vi "display_1s_stim_9s_ISI_CS1_CS2_no_trigger.vi"() -> ()   [LabVIEW 2019]
uses:
  <vilib>/Analysis/Matrix/Datatypes/RealMatrix.ctl
  <vilib>/Utility/file.llb/Write Delimited Spreadsheet (DBL).vi
  <vilib>/Analysis/Matrix/NI_Matrix.lvlib
panel:
  out "Num trials":u32=204
  out "ISI Time":dbl
  out "Stim TS":dbl
  out "Output":dbl[][](array[numeric])
  out "Output frame":T1
  out "Array temp1":T1
  out "Elapsed Time":dbl
  out "Display":bool=TRUE
  out "Trial":u32=1
  out "reward":dbl[](array[numeric])
  out "stim_id":dbl[](array[numeric])
  out "stim_loaded":dbl
  out "Timings":dbl[](array[numeric])
  out "Stimuli Loaded?":bool
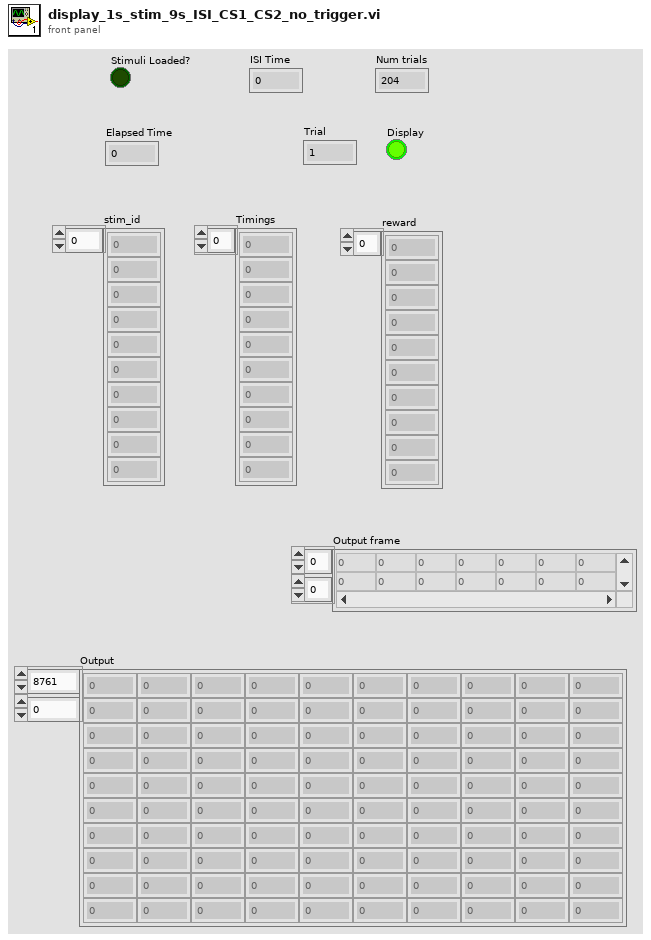
[diagram p1: front panel]
types:
  T1 = typedef "NI_Matrix.lvlib/RealMatrix.ctl" = dbl[][]
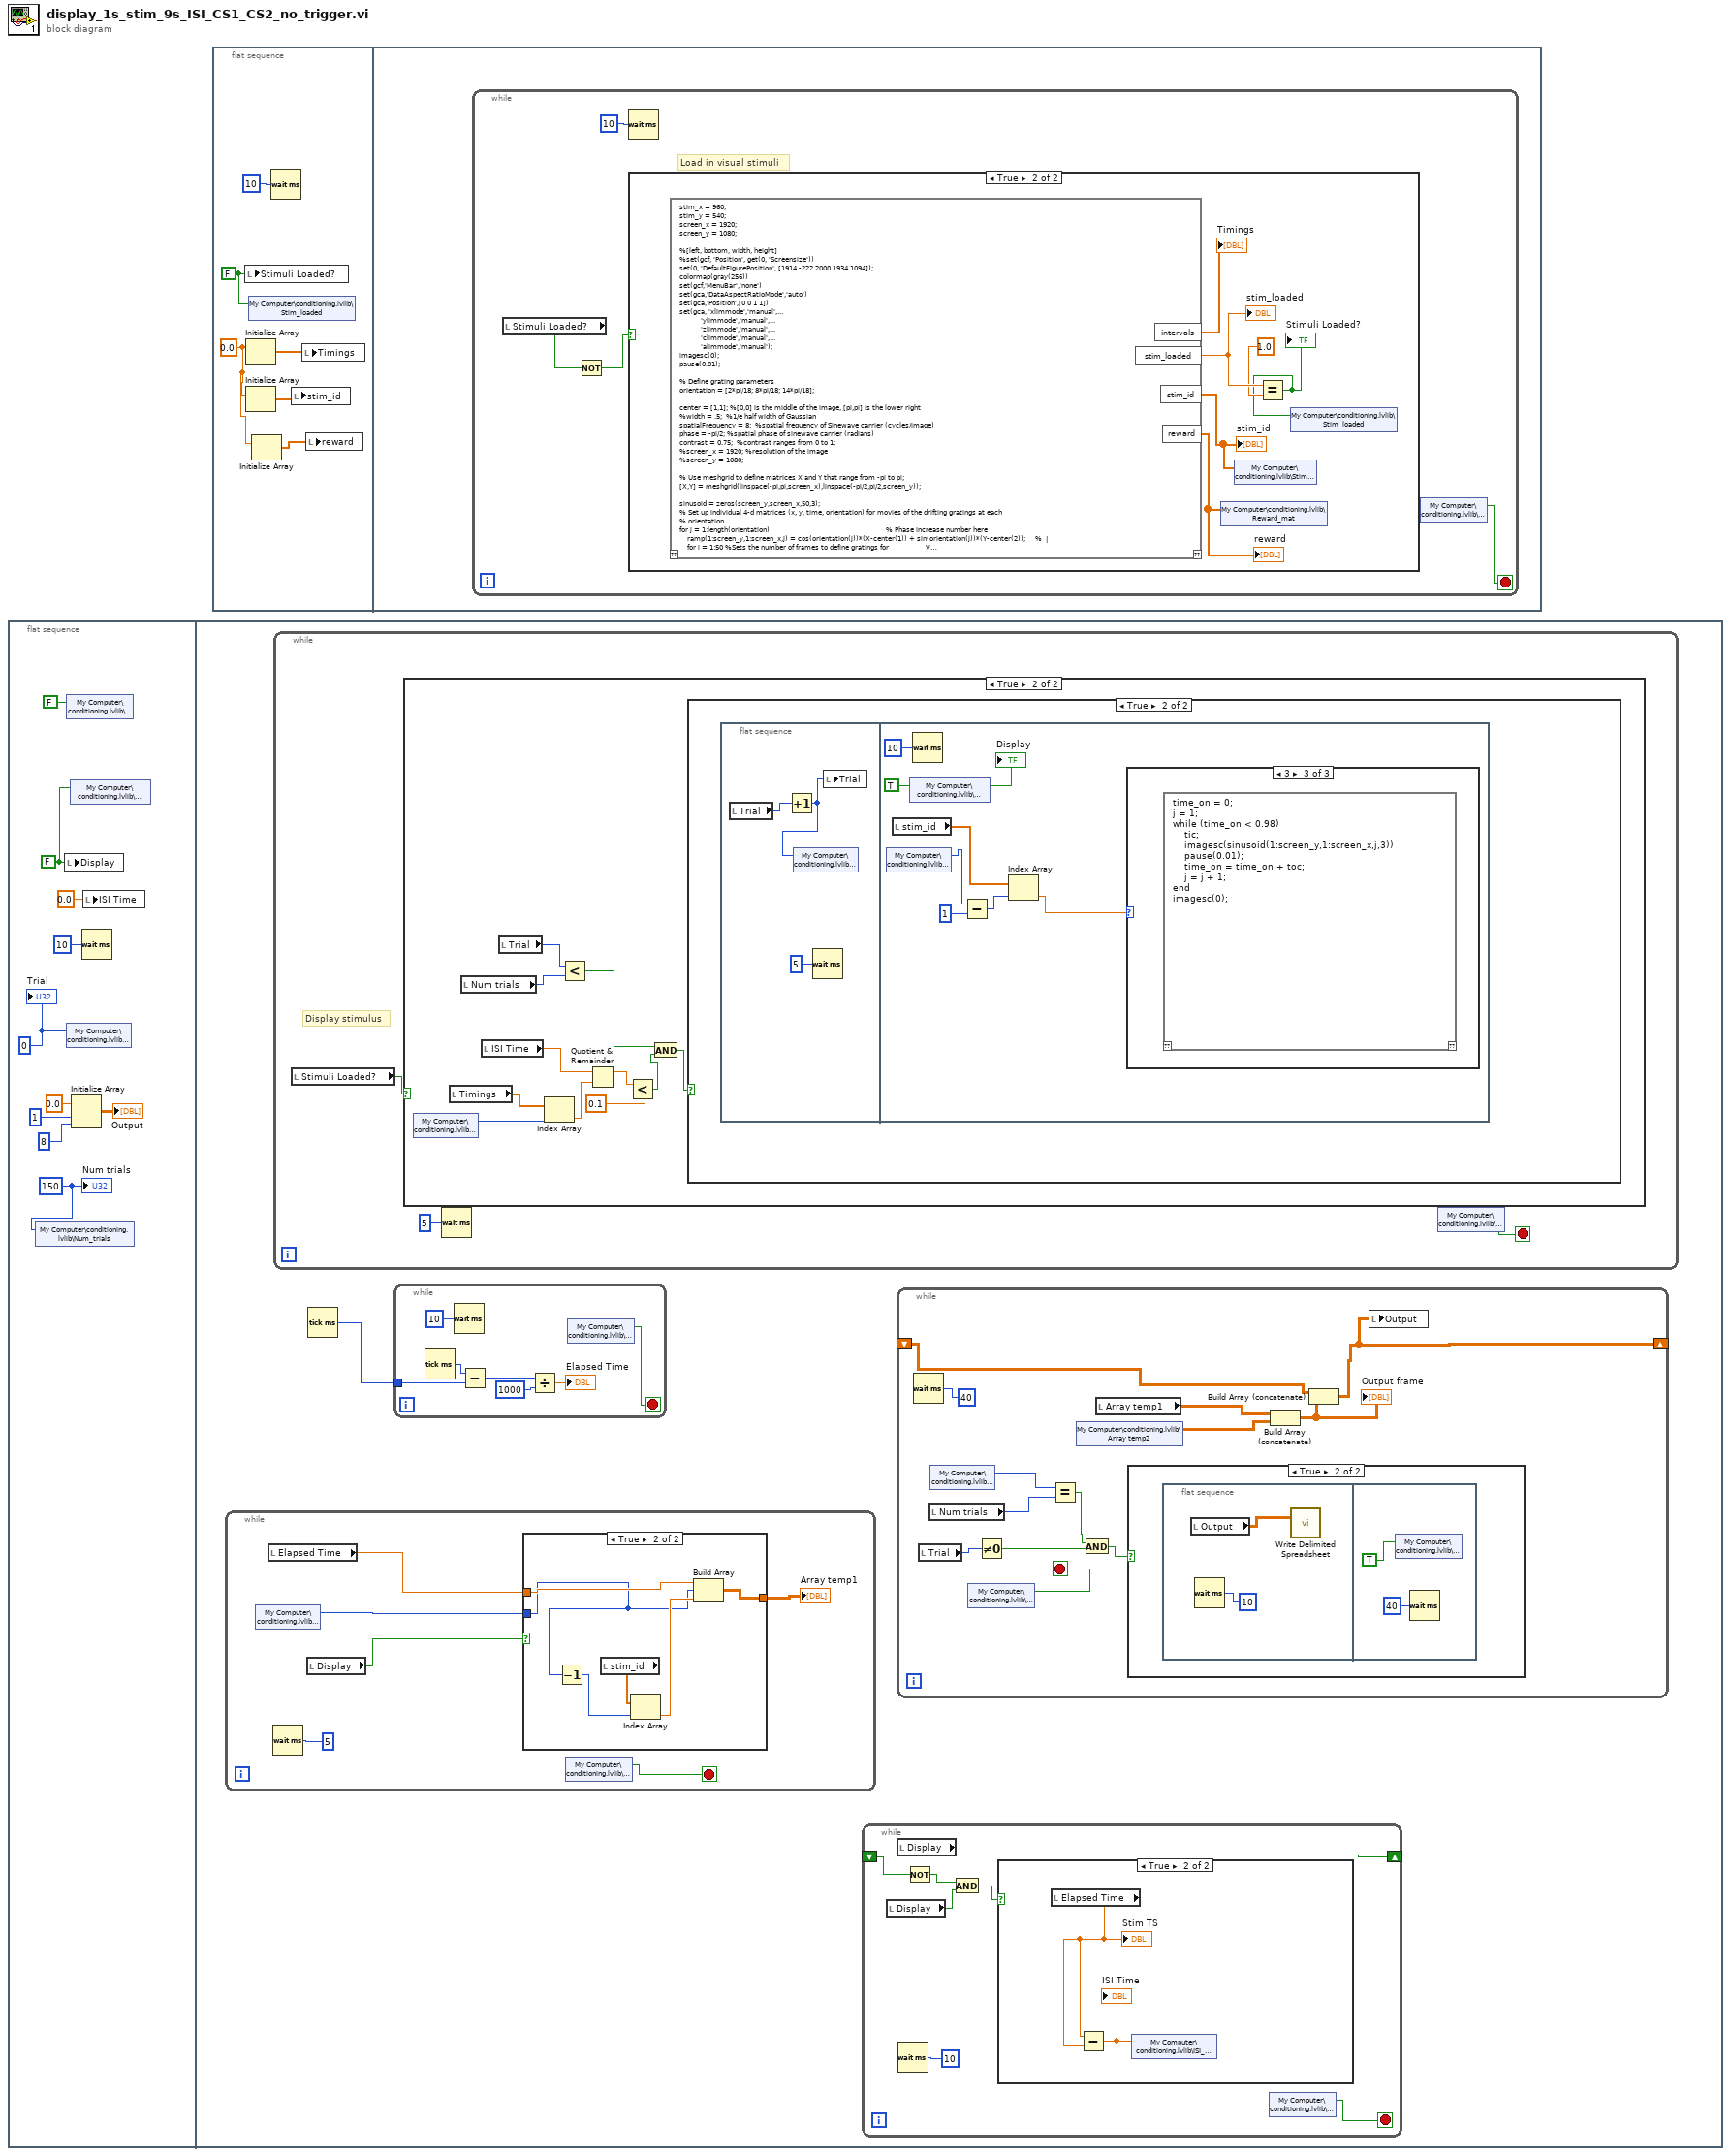
[diagram p0: block diagram]
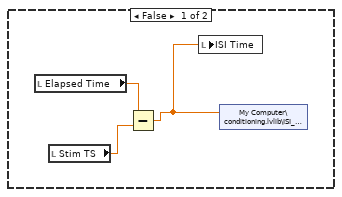
[diagram p3: hidden frame]
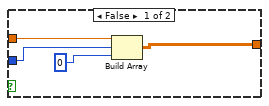
[diagram p4: hidden frame]
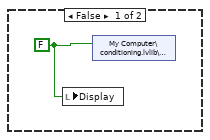
[diagram p7: hidden frame]
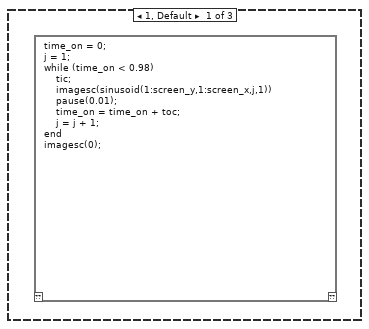
[diagram p8: hidden frame]
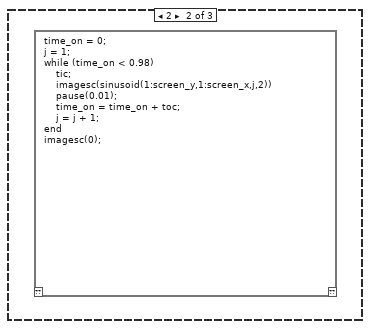
[diagram p9: hidden frame]
diagram:
  n1 = flat-sequence {
    frame #0 {
      w2 = u32 150
      w8 = FALSE ("Display")
      w10 = u32 0 ("Trial")
      n2 = shared-variable "My Computer\\conditioning.lvlib\\Num_trials"(w2) -> ()  [unwired: 1 in, 1 out]
      n3 = local write "Display"(w8) -> ()
      n4 = shared-variable "My Computer\\conditioning.lvlib\\Stop"(FALSE ("Stop")) -> ()  [unwired: 1 in, 1 out]
      n5 = shared-variable "My Computer\\conditioning.lvlib\\Trial"(w10) -> ()  [unwired: 1 in, 1 out]
      n6 = shared-variable "My Computer\\conditioning.lvlib\\Display"(w8) -> ()  [unwired: 1 in, 1 out]
      n7 = Initialize Array(0.0 ("element"), 1 ("dimension size"), 8 ("dimension size")) -> (→"Output":dbl[][])
      n8 = Wait (ms)(milliseconds to wait=u32 10) -> ()  [unwired: 1 out]
      n9 = local write "ISI Time"(0.0 ("ISI Time")) -> ()
      "Trial" <- w10
      "Num trials" <- w2
    }
    frame #1 {
      n10 = while {
        stop <- w24 stop-if-true
        n11 = shared-variable "My Computer\\conditioning.lvlib\\Trial"() -> (w26:u32)  [unwired: 1 in, 1 out]
        n12 = local read "Elapsed Time"() -> (w28:dbl)
        n13 = Wait (ms)(milliseconds to wait=u32 5) -> ()  [unwired: 1 out]
        n14 = local read "Display"() -> (w25:bool)
        n15 = case shown="True" w25 {
          tunnel: w26 -> [w32 w35]
          tunnel: w28 -> [w33 w37]
          tunnel: [w31 w38] -> w27
          frame False {
            n16 = Build Array(w33, w32, u32 0 ("milliseconds to wait")) -> (w31:T1)
          }
          frame True {
            n17 = Decrement(x=w35) -> (x-1=w34:u32)
            n18 = local read "stim_id"() -> (w39:dbl[])
            n19 = Index Array(array=w39, index=w34) -> (element=w36:dbl)
            n20 = Build Array(w37, w35, w36) -> (w38:T1)
          }
        }
        "Array temp1" <- w27
        n21 = shared-variable "My Computer\\conditioning.lvlib\\Stop"() -> (w24:bool)  [unwired: 1 in, 1 out]
      }
      n22 = while {
        stop <- w65 stop-if-true
        # "Display stimulus"
        n23 = local read "Stimuli Loaded?"() -> (w64:bool)
        n24 = case shown="True" w64 {
          frame False {
          }
          frame True {
            n25 = shared-variable "My Computer\\conditioning.lvlib\\Trial"() -> (w68:u32)  [unwired: 1 in, 1 out]
            n26 = local read "Timings"() -> (w75:dbl[])
            n27 = local read "Num trials"() -> (w67:u32)
            n28 = local read "ISI Time"() -> (w73:dbl)
            n29 = local read "Trial"() -> (w72:u32)
            n30 = Index Array(array=w75, index=w68) -> (element=w74:dbl)
            n31 = Less?(x=w72, y=w67) -> (x < y?=w71:bool)
            n32 = Quotient & Remainder(x=w73, y=w74) -> (x-y*floor(x/y)=w77:dbl)  [unwired: 1 out]
            n33 = Less?(x=w77, y=0.1) -> (x < y?=w70:bool)
            n34 = And(x=w71, y=w70) -> (x .and. y?=w69:bool)
            n35 = case shown="True" w69 {
              frame False {
                w78 = FALSE ("Display")
                n36 = local write "Display"(w78) -> ()
                n37 = shared-variable "My Computer\\conditioning.lvlib\\Display"(w78) -> ()  [unwired: 1 in, 1 out]
              }
              frame True {
                n38 = flat-sequence {
                  frame #0 {
                    n39 = local read "Trial"() -> (w80:u32)
                    n40 = Increment(x=w80) -> (x+1=w79:u32)
                    n41 = shared-variable "My Computer\\conditioning.lvlib\\Trial"(w79) -> ()  [unwired: 1 in, 1 out]
                    n42 = Wait (ms)(milliseconds to wait=u32 5) -> ()  [unwired: 1 out]
                    n43 = local write "Trial"(w79) -> ()
                  }
                  frame #1 {
                    w86 = TRUE ("Boolean")
                    n44 = shared-variable "My Computer\\conditioning.lvlib\\Trial"() -> (w84:u32)  [unwired: 1 in, 1 out]
                    n45 = local read "stim_id"() -> (w87:dbl[])
                    n46 = shared-variable "My Computer\\conditioning.lvlib\\Display"(w86) -> ()  [unwired: 1 in, 1 out]
                    n47 = Wait (ms)(milliseconds to wait=u32 10) -> ()  [unwired: 1 out]
                    n48 = Subtract(x=w84, y=u32 1) -> (x-y=w85:u32)
                    n49 = Index Array(array=w87, index=w85) -> (element=w82:dbl)
                    n50 = case shown="3" w82 {
                      frame 1, Default {
                        n51 = script code="time_on = 0;\nj = 1;\nwhile (time_on < 0.98)\n    tic;\n    imagesc(sinusoid(1:screen_y,1:screen_x,j,1))\n    pause(0.01);\n    time_on = time_on + toc;\n    j = j + 1;\nend\nimagesc(0);"() -> ()  [unwired: 1 in, 1 out]
                      }
                      frame 2 {
                        n52 = script code="time_on = 0;\nj = 1;\nwhile (time_on < 0.98)\n    tic;\n    imagesc(sinusoid(1:screen_y,1:screen_x,j,2))\n    pause(0.01);\n    time_on = time_on + toc;\n    j = j + 1;\nend\nimagesc(0);"() -> ()  [unwired: 1 in, 1 out]
                      }
                      frame 3 {
                        n53 = script code="time_on = 0;\nj = 1;\nwhile (time_on < 0.98)\n    tic;\n    imagesc(sinusoid(1:screen_y,1:screen_x,j,3))\n    pause(0.01);\n    time_on = time_on + toc;\n    j = j + 1;\nend\nimagesc(0);"() -> ()  [unwired: 1 in, 1 out]
                      }
                    }
                    "Display" <- w86
                  }
                }
              }
            }
          }
        }
        n54 = Wait (ms)(milliseconds to wait=u32 5) -> ()  [unwired: 1 out]
        n55 = shared-variable "My Computer\\conditioning.lvlib\\Stop"() -> (w65:bool)  [unwired: 1 in, 1 out]
      }
      n56 = Tick Count (ms)() -> (millisecond timer value=w11:u32)
      n57 = while {
        tunnel: w11 -> [w43]
        stop <- w40 stop-if-true
        n58 = Tick Count (ms)() -> (millisecond timer value=w44:u32)
        n59 = Wait (ms)(milliseconds to wait=u32 10) -> ()  [unwired: 1 out]
        n60 = Subtract(x=w44, y=w43) -> (x-y=w41:u32)
        n61 = Divide(x=w41, y=u32 1000) -> (x/y=→"Elapsed Time":dbl)
        n62 = shared-variable "My Computer\\conditioning.lvlib\\Stop"() -> (w40:bool)  [unwired: 1 in, 1 out]
      }
      n63 = while {
        shift-right: [w16] -> _
        shift-left: _ -> [w15]
        stop <- w18 stop-if-true
        n64 = local read "Display"() -> (w13:bool)
        n65 = local read "Display"() -> (w16:bool)
        n66 = Wait (ms)(milliseconds to wait=u32 10) -> ()  [unwired: 1 out]
        n67 = Not(x=w15) -> (.not. x?=w14:bool)
        n68 = And(x=w14, y=w13) -> (x .and. y?=w12:bool)
        n69 = case shown="True" w12 {
          frame False {
            n70 = local read "Elapsed Time"() -> (w19:dbl)
            n71 = local read "Stim TS"() -> (w21:dbl)
            n72 = Subtract(x=w19, y=w21) -> (x-y=w20:dbl)
            n73 = local write "ISI Time"(w20) -> ()
            n74 = shared-variable "My Computer\\conditioning.lvlib\\ISI_Time"(w20) -> ()  [unwired: 1 in, 1 out]
          }
          frame True {
            n75 = local read "Elapsed Time"() -> (w22:dbl)
            "Stim TS" <- w22
            n76 = Subtract(x=w22, y=w22) -> (x-y=w23:dbl)
            "ISI Time" <- w23
            n77 = shared-variable "My Computer\\conditioning.lvlib\\ISI_Time"(w23) -> ()  [unwired: 1 in, 1 out]
          }
        }
        n78 = shared-variable "My Computer\\conditioning.lvlib\\Stop"() -> (w18:bool)  [unwired: 1 in, 1 out]
      }
      n79 = while {
        shift-right: [w56] -> _
        shift-left: _ -> [w57]
        stop <- w59 stop-if-true
        n80 = Wait (ms)(milliseconds to wait=u32 40) -> ()  [unwired: 1 out]
        n81 = local read "Trial"() -> (w49:u32)
        n82 = local read "Num trials"() -> (w51:u32)
        n83 = shared-variable "My Computer\\conditioning.lvlib\\Trial"() -> (w52:u32)  [unwired: 1 in, 1 out]
        n84 = shared-variable "My Computer\\conditioning.lvlib\\Stop"() -> (w59:bool)  [unwired: 1 in, 1 out]
        n85 = Not Equal To 0?(x=w49) -> (x != 0?=w48:bool)
        n86 = Equal?(x=w52, y=w51) -> (x = y?=w50:bool)
        n87 = shared-variable "My Computer\\conditioning.lvlib\\Array temp2"() -> (w54:dbl[][])  [unwired: 1 in, 1 out]
        n88 = And(x=w50, y=w48) -> (x .and. y?=w47:bool)
        n89 = local read "Array temp1"() -> (w55:T1)
        n90 = case shown="True" w47 {
          frame False {
          }
          frame True {
            n91 = flat-sequence {
              frame #0 {
                n92 = local read "Output"() -> (w61:dbl[][])
                n93 = Wait (ms)(milliseconds to wait=u32 10) -> ()  [unwired: 1 out]
                n94 = call-poly <vilib>:"Write Delimited Spreadsheet.vi"("2D data"=w61) -> ()  [unwired: 13 in, 2 out]
              }
              frame #1 {
                n95 = shared-variable "My Computer\\conditioning.lvlib\\Stop"(TRUE) -> ()  [unwired: 1 in, 1 out]
                n96 = Wait (ms)(milliseconds to wait=u32 40) -> ()  [unwired: 1 out]
              }
            }
          }
        }
        n97 = Build Array (concatenate)(w55, w54) -> (w53:T1)
        "Output frame" <- w53
        n98 = Build Array (concatenate) ("Build Matrix")(w57, w53) -> (w56:T1)
        n99 = local write "Output"(w56) -> ()
      }
    }
  }
  n100 = flat-sequence {
    frame #0 {
      w91 = 0.0 ("element")
      w89 = FALSE ("Stimuli Loaded?")
      n101 = local write "Stimuli Loaded?"(w89) -> ()
      n102 = Initialize Array(w91) -> (w93:dbl[])  [unwired: 1 in]
      n103 = Initialize Array(w91) -> (w92:dbl[])  [unwired: 1 in]
      n104 = shared-variable "My Computer\\conditioning.lvlib\\Stim_loaded"(w89) -> ()  [unwired: 1 in, 1 out]
      n105 = Initialize Array(w91) -> (w90:dbl[])  [unwired: 1 in]
      n106 = Wait (ms)(milliseconds to wait=u32 10) -> ()  [unwired: 1 out]
      n107 = local write "stim_id"(w92) -> ()
      n108 = local write "Timings"(w93) -> ()
      n109 = local write "reward"(w90) -> ()
    }
    frame #1 {
      n110 = while {
        stop <- w97 stop-if-true
        # "Load in visual stimuli"
        n111 = local read "Stimuli Loaded?"() -> (w96:bool)
        n112 = Not(x=w96) -> (.not. x?=w95:bool)
        n113 = Wait (ms)(milliseconds to wait=u32 10) -> ()  [unwired: 1 out]
        n114 = case shown="True" w95 {
          frame False {
          }
          frame True {
            n115 = script code="stim_x = 960;\nstim_y = 540;\nscreen_x = 1920;\nscreen_y = 1080;\n\n%[left, bottom, width, height]\n%set(gcf, 'Position', get(0, 'Screensize'))\nset(0, 'DefaultFigurePosition', [1914 -222.2000 1934 1094]);\ncolormap(gray(256))\nset(gcf,'MenuBar','none')\nset(gca,'DataAspectRatioMode','auto')\nset(gca,'Position',[0 0 1 1])\nset(gca, 'xlimmode','manual',...\n           'ylimmode','manual',...\n           'zlimmode','manual',...\n           'climmode','manual',...\n           'alimmode','manual');\nimagesc(0);\npause(0.01);\n\n% Define grating parameters\norientation = [2*pi/18; 8*pi/18; 14*pi/18];\n\ncenter = [1,1]; %[0,0] is the middle of the image, [pi,pi] is the lower right\n%width = .5;  %1/e half width of Gaussian\nspatialFrequency = 8;  %spatial frequency of Sinewave carrier (cycles/image)\nphase = -pi/2; %spatial phase of sinewave carrier (radians)\ncontrast = 0.75;  %contrast ranges from 0 to 1;\n%screen_x = 1920; %resolution of the image  \n%screen_y = 1080;\n\n% Use meshgrid to define matrices X and Y that range from -pi to pi;\n[X,Y] = meshgrid(linspace(-pi,pi,screen_x),linspace(-pi/2,pi/2,screen_y));\n\nsinusoid = zeros(screen_y,screen_x,50,3);\n% Set up individual 4-d matrices (x, y, time, orientation) for movies of the drifting gratings at each\n% orientation\nfor j = 1:length(orientation)                                                            % Phase increase number here\n    ramp(1:screen_y,1:screen_x,j) = cos(orientation(j))*(X-center(1)) + sin(orientation(j))*(Y-center(2));     %  |\n    for i = 1:50 %Sets the number of frames to define gratings for                   V\n       sinusoid(1:screen_y,1:screen_x,i,j) = contrast*sin(spatialFrequency*ramp(1:screen_y,1:screen_x,j)-...\n           (phase+(2*pi*(i-1)*(-30)/360))); %Number before '/360' sets the phase increase\n    end\nend\n\nintervals = [ones(1,41)*10 ones(1,41)*11 ones(1,41)*12 ones(1,41)*13 ones(1,40)*14];\nintervals = intervals(randperm(204));\nrand_idx = randperm(204);\nstim_id = [ones(1,102)*1 ones(1,102)*2];\nstim_id = stim_id(rand_idx);\nreward = [ones(1,102)*1 ones(1,102)*1];\nreward = reward(rand_idx);\n\nstim_loaded = 1;" ("Script Node")() -> ("stim_loaded"=w104:dbl, "intervals"=→"Timings":dbl[], "stim_id"=w99:dbl[], "reward"=w101:dbl[])  [unwired: 1 in, 1 out]
            "stim_loaded" <- w104
            "stim_id" <- w99
            "reward" <- w101
            n116 = shared-variable "My Computer\\conditioning.lvlib\\Reward_mat"(w101) -> ()  [unwired: 1 in, 1 out]
            n117 = shared-variable "My Computer\\conditioning.lvlib\\Stim_ID"(w99) -> ()  [unwired: 1 in, 1 out]
            n118 = Equal?(x=w104, y=1.0) -> (x = y?=w100:bool)
            "Stimuli Loaded?" <- w100
            n119 = shared-variable "My Computer\\conditioning.lvlib\\Stim_loaded"(w100) -> ()  [unwired: 1 in, 1 out]
          }
        }
        n120 = shared-variable "My Computer\\conditioning.lvlib\\Stop"() -> (w97:bool)  [unwired: 1 in, 1 out]
      }
    }
  }
